vi "IP Available.vi"(3 "dot notation? (T)":bool=TRUE) -> (4 "IPs availables":i32, 5 "IP/Domain":string[](array[string]))   [LabVIEW 2021, in "IP addresses.lvlib"]
uses:
  IP addresses.lvlib
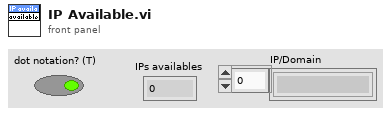
[diagram p1: front panel]
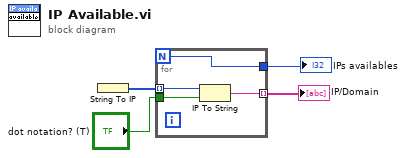
[diagram p0: block diagram]
diagram:
  n1 = String To IP() -> (0:w3:u32[])  [unwired: 1 in]
  n2 = for {
    N -> [w5]
    tunnel: [w8] -> w4 mode=indexing
    tunnel: w3 -> [w7] mode=indexing
    tunnel: "dot notation? (T)" -> [w6]
    tunnel: [w5] -> w1
    n3 = IP To String(1:w6, 2:w7) -> (0:w8:string)
  }
  "IP/Domain" <- w4
  "IPs availables" <- w1
